vi "PS4 Controller Event Structure.vi"() -> ()   [LabVIEW 2011, in "LVH-PS4.lvlib"]
uses:
  LVH-PS4.lvlib
panel:
  in  "Device Index":i32
  in  "Stop Button":bool
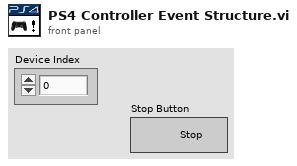
[diagram p1: front panel]
types:
  T1 = typedef "LVH-PS4.lvlib/PS4 Controller Ref.ctl" = cluster{"Controller Ref":refnum<k1>, "PS4 Events Ref":refnum<event-registration>, "Worker Ref":refnum<vi>}
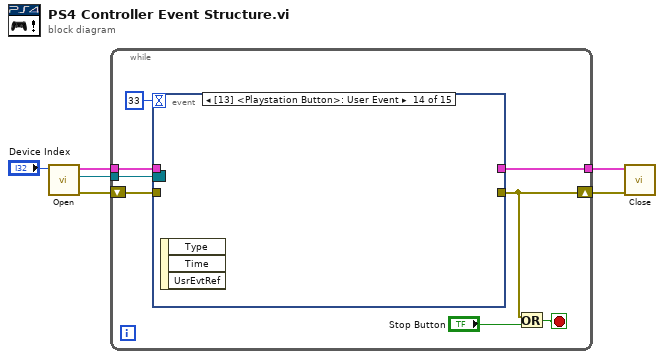
[diagram p0: block diagram]
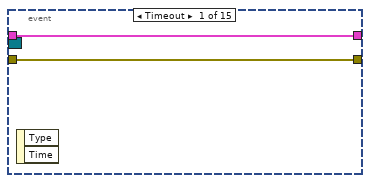
[diagram p2: hidden frame]
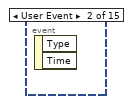
[diagram p3: hidden frame]
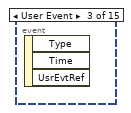
[diagram p4: hidden frame]
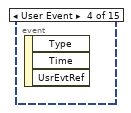
[diagram p5: hidden frame]
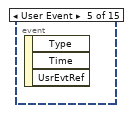
[diagram p6: hidden frame]
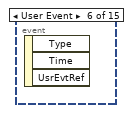
[diagram p7: hidden frame]
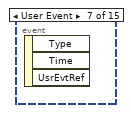
[diagram p8: hidden frame]
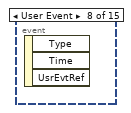
[diagram p9: hidden frame]
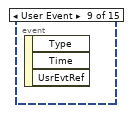
[diagram p10: hidden frame]
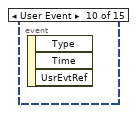
[diagram p11: hidden frame]
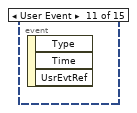
[diagram p12: hidden frame]
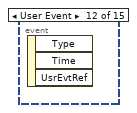
[diagram p13: hidden frame]
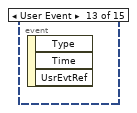
[diagram p14: hidden frame]
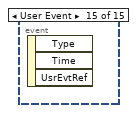
[diagram p15: hidden frame]
diagram:
  n1 = call "Open.vi"("Device Index"="Device Index") -> ("Error Out"=w4:errorcluster, "PS4 Event Refs"=w2:refnum<event-registration>, "PS4 Controller Ref"=w3:T1)  [unwired: 8 in]
  n2 = while {
    shift-right: [w10] -> w6
    shift-left: w4 -> [w13]
    tunnel: w3 -> [w14]
    tunnel: [w9] -> w5
    tunnel: w2 -> [w7]
    stop <- w12 stop-if-true
    n3 = event shown="[13] <Playstation Button>: User Event" {
      selector: w7 -> [_ _ _ _ _ _ _ _ _ _ _ _ _ _ _]
      dyn-events: _ -> [_ _ _ _ _ _ _ _ _ _ _ _ _ _ _]
      timeout: 33 -> [_ _ _ _ _ _ _ _ _ _ _ _ _ _ _]
      tunnel: w14 -> [w16 _ _ _ _ _ _ _ _ _ _ _ _ _ _]
      tunnel: w13 -> [w15 _ _ _ _ _ _ _ _ _ _ _ _ _ _]
      tunnel: [w15 _ _ _ _ _ _ _ _ _ _ _ _ _ _] -> w10
      tunnel: [w16 _ _ _ _ _ _ _ _ _ _ _ _ _ _] -> w9
      event Timeout {
        n4 = event-data() -> ()  [unwired: 1 in, 2 out]
      }
      event User Event {
        n5 = event-data() -> ()  [unwired: 1 in, 2 out]
      }
      event User Event {
        n6 = event-data() -> ()  [unwired: 1 in, 3 out]
      }
      event User Event {
        n7 = event-data() -> ()  [unwired: 1 in, 3 out]
      }
      event User Event {
        n8 = event-data() -> ()  [unwired: 1 in, 3 out]
      }
      event User Event {
        n9 = event-data() -> ()  [unwired: 1 in, 3 out]
      }
      event User Event {
        n10 = event-data() -> ()  [unwired: 1 in, 3 out]
      }
      event User Event {
        n11 = event-data() -> ()  [unwired: 1 in, 3 out]
      }
      event User Event {
        n12 = event-data() -> ()  [unwired: 1 in, 3 out]
      }
      event User Event {
        n13 = event-data() -> ()  [unwired: 1 in, 3 out]
      }
      event User Event {
        n14 = event-data() -> ()  [unwired: 1 in, 3 out]
      }
      event User Event {
        n15 = event-data() -> ()  [unwired: 1 in, 3 out]
      }
      event User Event {
        n16 = event-data() -> ()  [unwired: 1 in, 3 out]
      }
      event User Event {
        n17 = event-data() -> ()  [unwired: 1 in, 3 out]
      }
      event User Event {
        n18 = event-data() -> ()  [unwired: 1 in, 3 out]
      }
    }
    n19 = Or(x=w10, y="Stop Button") -> (x .or. y?=w12:bool)
  }
  n20 = call "Close.vi"("Error In"=w6, "PS4 Controller Ref"=w5) -> ()  [unwired: 9 in, 1 out]
